vi "Translator OTA Functions.vi"(0 "Input":variant, 11 "error in (no error)":errorcluster) -> (4 "Output":variant, 15 "error out":errorcluster)   [LabVIEW 2014, in "ESP8266 WiFi Wrapper.lvlib"]
doc: "An example of how to create the Translator to convert the LabVIEW VIs to Arduino C code."
uses:
  ESP8266 WiFi Wrapper.lvlib
panel:
  out "Outputs":string[](array[string])
  out "Inputs":string[](array[string])
  out "Output Datatypes":string[](array[string])
  out "Input Datatypes":string[](array[string])
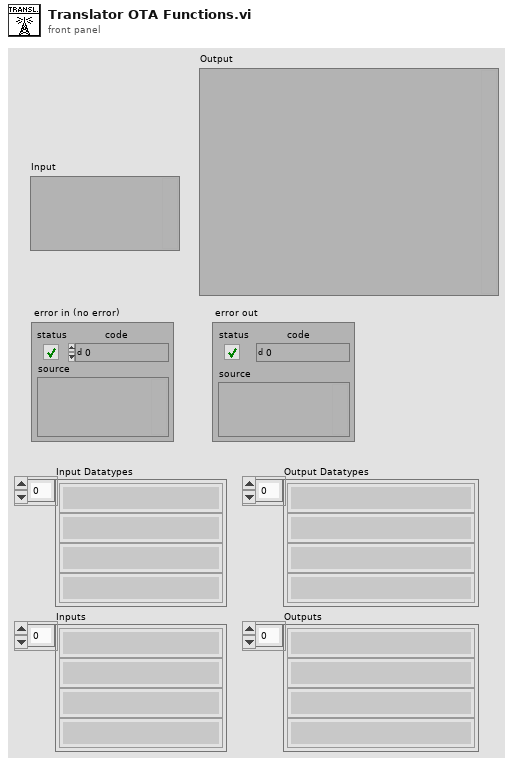
[diagram p1: front panel]
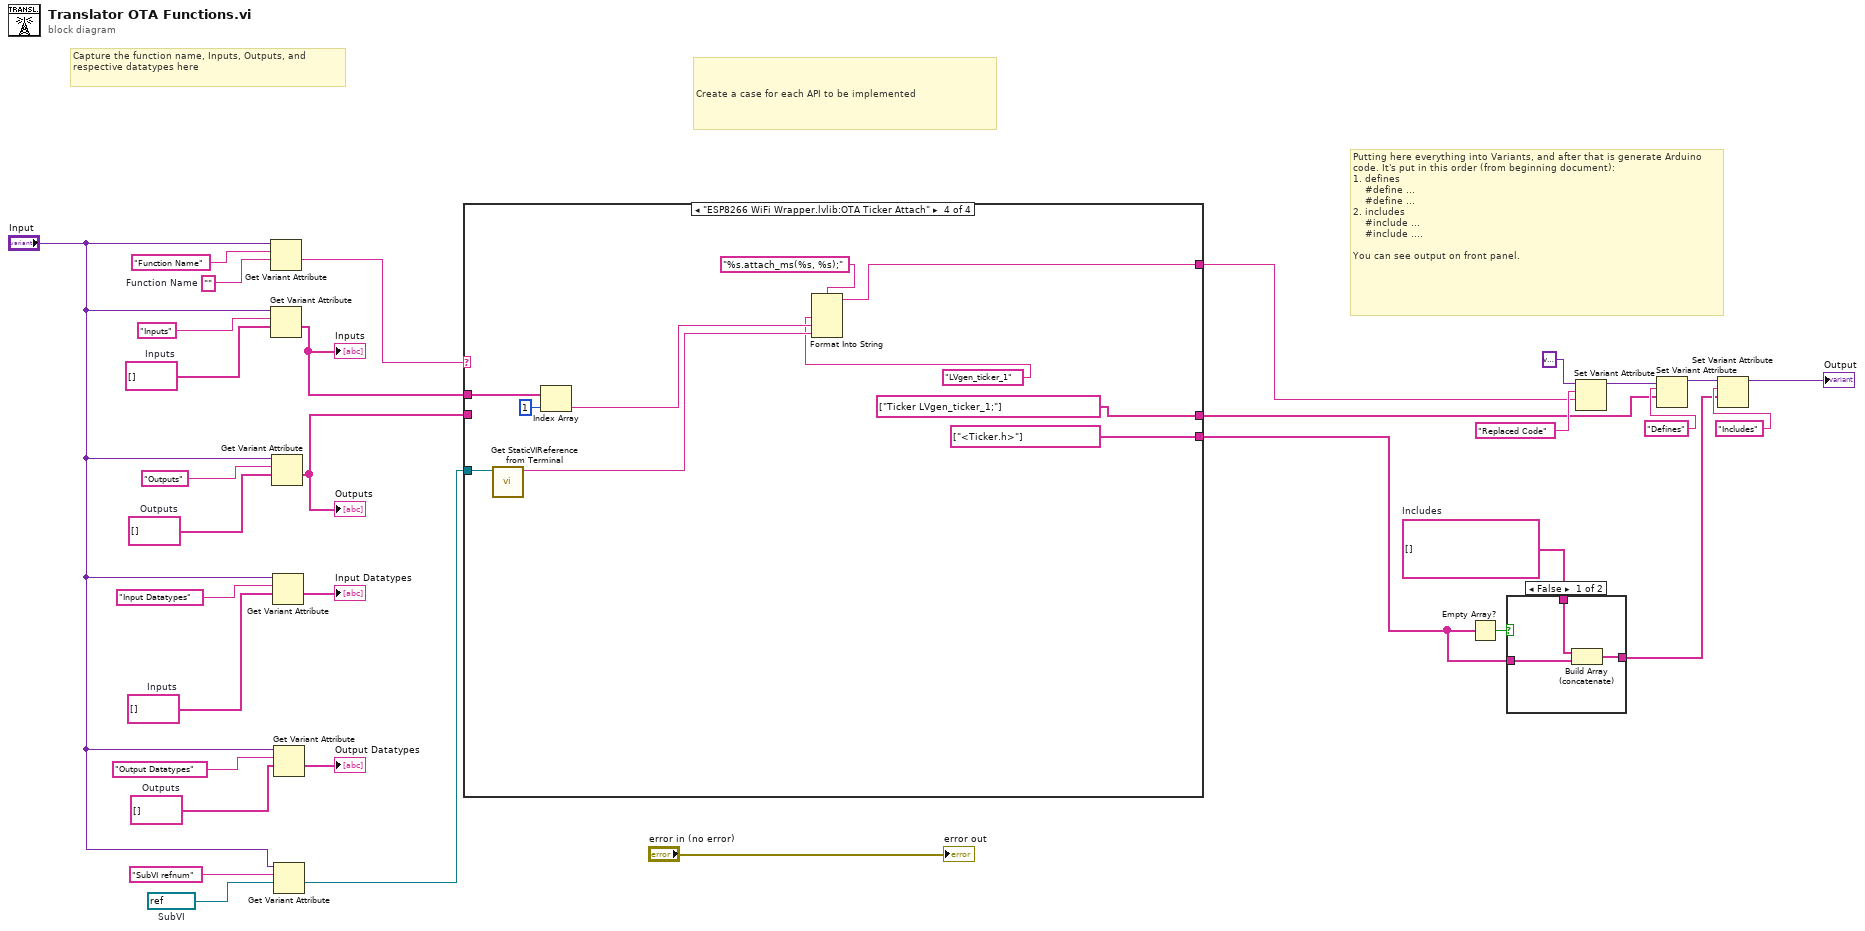
[diagram p0: block diagram]
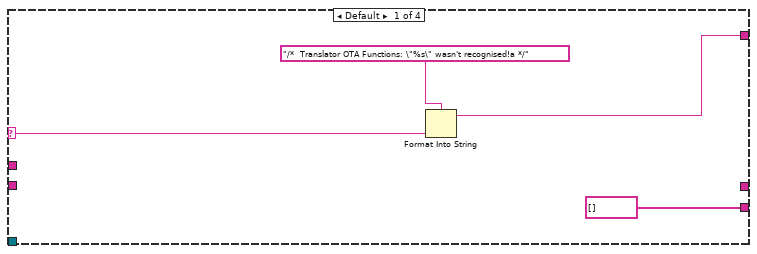
[diagram p3: hidden frame]
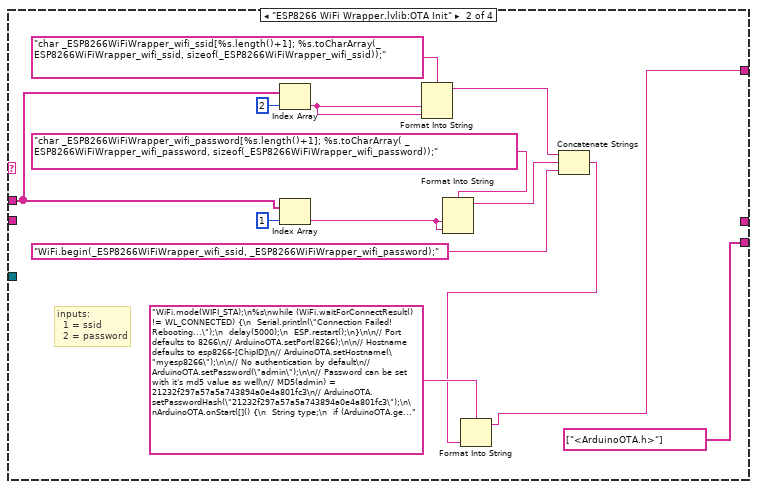
[diagram p4: hidden frame]
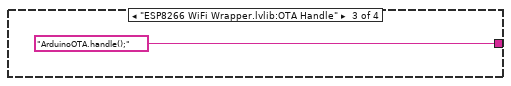
[diagram p5: hidden frame]
diagram:
  w1 = refnum<vi> refnum  # SubVI
  w22 = string[] []  # Outputs
  w23 = string[] []  # Inputs
  w8 = string[] []  # Includes
  w29 = string[] []  # Outputs
  w30 = string[] []  # Inputs
  w31 = ""  # Function Name
  # "Capture the function name, Inputs, Outputs, and respective datatypes here"
  # "Putting here everything into Variants, and after that is generate Arduino code. It's put in this order (from beginning document):\n1. defines\n    #define ...\n    #define ...\n2. includes\n    #include ...\n    #include ....\n\nYou can see output on front panel."
  # "Create a case for each API to be implemented"
  n1 = Get Variant Attribute(Variant="Input", name="Function Name", default value (empty Variant)=w31) -> (value=w14:string)  [unwired: 1 in, 3 out]
  n2 = Get Variant Attribute(Variant="Input", name="Inputs", default value (empty Variant)=w30) -> (value=w13:string[])  [unwired: 1 in, 3 out]
  "Inputs" <- w13
  n3 = Get Variant Attribute(Variant="Input", name="Outputs", default value (empty Variant)=w29) -> (value=w12:string[])  [unwired: 1 in, 3 out]
  "Outputs" <- w12
  n4 = Get Variant Attribute(Variant="Input", name="Input Datatypes", default value (empty Variant)=w23) -> (value=→"Input Datatypes":string[])  [unwired: 1 in, 3 out]
  n5 = Get Variant Attribute(Variant="Input", name="Output Datatypes", default value (empty Variant)=w22) -> (value=→"Output Datatypes":string[])  [unwired: 1 in, 3 out]
  n6 = Get Variant Attribute(Variant="Input", name="SubVI refnum", default value (empty Variant)=w1) -> (value=w3:refnum<vi>)  [unwired: 1 in, 3 out]
  n7 = case shown="\"ESP8266 WiFi Wrapper.lvlib:OTA Ticker Attach\"" w14 {
    selector: w14 -> [w37 _ _ _]
    tunnel: w13 -> [_ w41 _ w58]
    tunnel: w12 -> [_ _ _ _]
    tunnel: [w36 w38 "ArduinoOTA.handle();" w56] -> w11
    tunnel: [string[] [] string[] ["<ArduinoOTA.h>"] _ string[] ["<Ticker.h>"]] -> w6
    tunnel: [_ _ _ string[] ["Ticker LVgen_ticker_1;"]] -> w5
    tunnel: w3 -> [_ _ _ w60]
    frame Default {
      n8 = Format Into String(format string="/*  Translator OTA Functions: \"%s\" wasn't recognised!a */", w37) -> (resulting string=w36:string)  [unwired: 2 in, 1 out]
    }
    frame "ESP8266 WiFi Wrapper.lvlib:OTA Init" {
      # "inputs:\n  1 = ssid\n  2 = password"
      n9 = Index Array(array=w41, index=2) -> (element=w43:string)
      n10 = Index Array(array=w41, index=1) -> (element=w42:string)
      n11 = Format Into String(format string="char _ESP8266WiFiWrapper_wifi_ssid[%s.length()+1]; %s.toCharArray(_ESP8266WiFiWrapper_wifi_ssid, sizeof(_ESP8266WiFiWrapper_wifi_ssid));" ("name"), w43, w43) -> (resulting string=w46:string)  [unwired: 2 in, 1 out]
      n12 = Format Into String(format string="char _ESP8266WiFiWrapper_wifi_password[%s.length()+1]; %s.toCharArray( _ESP8266WiFiWrapper_wifi_password, sizeof(_ESP8266WiFiWrapper_wifi_password));" ("name"), w42, w42) -> (resulting string=w45:string)  [unwired: 2 in, 1 out]
      n13 = Concatenate Strings(w46, w45, "WiFi.begin(_ESP8266WiFiWrapper_wifi_ssid, _ESP8266WiFiWrapper_wifi_password);" ("name")) -> (w39:string)
      n14 = Format Into String(format string="WiFi.mode(WIFI_STA);\n%s\nwhile (WiFi.waitForConnectResult() != WL_CONNECTED) {\n  Serial.println(\"Connection Failed! Rebooting...\");\n  delay(5000);\n  ESP.restart();\n}\n\n// Port defaults to 8266\n// ArduinoOTA.setPort(8266);\n\n// Hostname defaults to esp8266-[ChipID]\n// ArduinoOTA.setHostname(\"myesp8266\");\n\n// No authentication by default\n// ArduinoOTA.setPassword(\"admin\");\n\n// Password can be set with it's md5 value as well\n// MD5(admin) = 21232f297a57a5a743894a0e4a801fc3\n// ArduinoOTA.setPasswordHash(\"21232f297a57a5a743894a0e4a801fc3\");\n\nArduinoOTA.onStart([]() {\n  String type;\n  if (ArduinoOTA.getCommand() == U_FLASH) {\n    type = \"sketch\";\n  } else { // U_SPIFFS\n    type = \"filesystem\";\n  }\n\n  // NOTE: if updating SPIFFS this would be the place to unmount SPIFFS using SPIFFS.end()\n  Serial.println(\"Start updating \" + type);\n});\nArduinoOTA.onEnd([]() {\n  Serial.println(\"\");\n  Serial.println(\"End\");\n});\nArduinoOTA.onProgress([](unsigned int progress, unsigned int total) {\n  Serial.printf(\"Progress: \\%u\\%\\%\\\\r\", (progress / (total / 100)));\n});\nArduinoOTA.onError([](ota_error_t error) {\n  Serial.printf(\"Error[\\%u]: \", error);\n  if (error == OTA_AUTH_ERROR) {\n    Serial.println(\"Auth Failed\");\n  } else if (error == OTA_BEGIN_ERROR) {\n    Serial.println(\"Begin Failed\");\n  } else if (error == OTA_CONNECT_ERROR) {\n    Serial.println(\"Connect Failed\");\n  } else if (error == OTA_RECEIVE_ERROR) {\n    Serial.println(\"Receive Failed\");\n  } else if (error == OTA_END_ERROR) {\n    Serial.println(\"End Failed\");\n  }\n});\nArduinoOTA.begin();\nSerial.println(\"Ready\");\nSerial.print(\"IP address: \");\nSerial.println(WiFi.localIP());", w39) -> (resulting string=w38:string)  [unwired: 2 in, 1 out]
    }
    frame "ESP8266 WiFi Wrapper.lvlib:OTA Handle" {
    }
    frame "ESP8266 WiFi Wrapper.lvlib:OTA Ticker Attach" {
      n15 = call <vilib>:"Get StaticVIReference from Terminal.vi"("SubVI in"=w60) -> ("String"=w54:string)  [unwired: 10 in]
      n16 = Index Array(array=w58, index=1) -> (element=w55:string)
      n17 = Format Into String(format string="%s.attach_ms(%s, %s);", "LVgen_ticker_1" ("input 1"), w55, w54) -> (resulting string=w56:string)  [unwired: 2 in, 1 out]
    }
  }
  n18 = Empty Array?(array=w6) -> (empty?=w7:bool)
  n19 = case shown="False" w7 {
    tunnel: w6 -> [w63 _]
    tunnel: [w65 w66] -> w9
    tunnel: w8 -> [w64 w66]
    frame False {
      n20 = Build Array (concatenate)(w64, w63) -> (w65:string[])
    }
    frame True {
    }
  }
  n21 = Set Variant Attribute(Variant=variant ("variant"), name="Replaced Code", value=w11) -> (Variant out=w17:variant)  [unwired: 1 in, 2 out]
  n22 = Set Variant Attribute(Variant=w17, name="Defines", value=w5) -> (Variant out=w16:variant)  [unwired: 1 in, 2 out]
  n23 = Set Variant Attribute(Variant=w16, name="Includes", value=w9) -> (Variant out=→"Output":variant)  [unwired: 1 in, 2 out]
  "error out" <- "error in (no error)"
